vi "getRGBInt.vi"(8 "Fiber Num":i32, 10 "Error":bool, 11 "VISA resource name":refnum<visa-resource-name>="ASRL13::INSTR") -> (0 "Green":u8, 1 "Red":u8, 2 "Error":bool, 3 "dup VISA resource name":refnum<visa-resource-name>="ASRL13::INSTR", 4 "Blue":u8, 6 "Intensity":u32)   [LabVIEW 2020, in "Library Instrument & Equipement.lvlib" / "Library LED Analyser.lvlib"]
uses:
  Library LED Analyser.lvlib
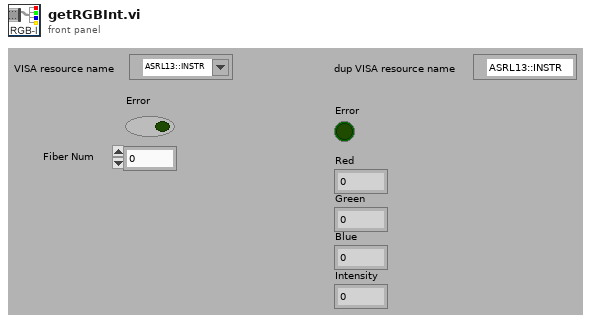
[diagram p1: front panel]
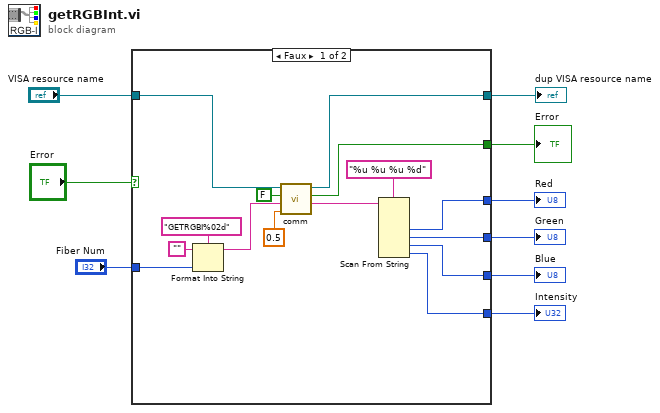
[diagram p0: block diagram]
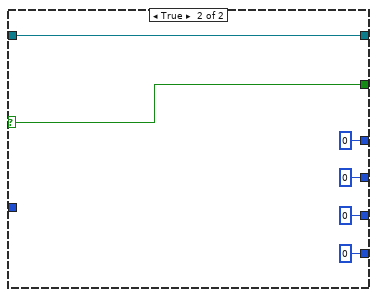
[diagram p2: hidden frame]
diagram:
  n1 = case shown="Faux" "Error" {
    selector: "Error" -> [_ w29]
    tunnel: "VISA resource name" -> [w24 w30]
    tunnel: "Fiber Num" -> [w21 _]
    tunnel: [w17 0] -> w7
    tunnel: [w16 0] -> w6
    tunnel: [w15 0] -> w5
    tunnel: [w14 0] -> w4
    tunnel: [w13 w30] -> w2
    tunnel: [w12 w29] -> w1
    frame False {
      n2 = Format Into String(format string="GETRGBI%02d" ("Substring"), initial string="", w21) -> (resulting string=w20:string)  [unwired: 1 in, 1 out]
      n3 = call "comm.vi"("Timeout (s)"=0.5, "Command"=w20, "Error"=FALSE, "VISA resource name"=w24) -> ("Response"=w19:string, "Error"=w12:bool, "dup VISA resource name"=w13:refnum<visa-resource-name>)  [unwired: 2 in, 1 out]
      n4 = Scan From String(format string="%u %u %u %d", input string=w19) -> (output 1=w17:u32, output 2=w16:u32, output 3=w15:u32, output 4=w14:i32)  [unwired: 6 in, 3 out]
    }
    frame True {
    }
  }
  "Red" <- w7
  "Intensity" <- w4
  "Green" <- w6
  "Blue" <- w5
  "Error" <- w1
  "dup VISA resource name" <- w2
